vi "总磷总氮量程写入.vi"(7 "error in (no error)":errorcluster caption="错误输入（无错误）", 9 "量程参数写入":T1, 10 "测量参数":enum16{"总磷", "总氮"}(ring)) -> (0 "error out":errorcluster caption="错误输出")   [LabVIEW 2016, in "斯坦道总磷.lvlib"]
panel:
  out "输出数组":u16[](array[numeric]) format="%04x"
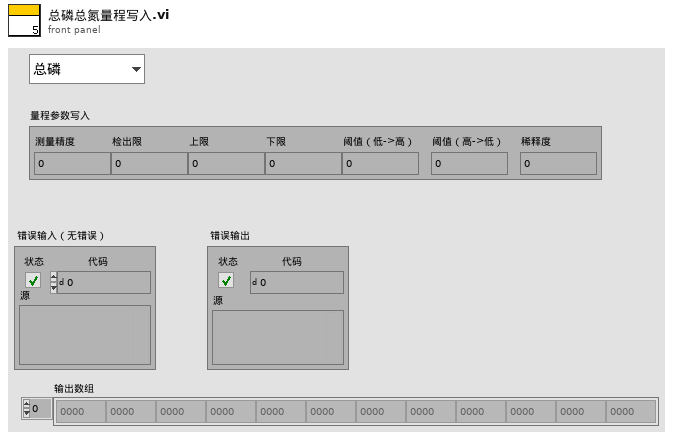
[diagram p1: front panel]
types:
  T1 = cluster{"测量精度":u16, "检出限":dbl, "上限":dbl, "下限":dbl, "阈值（低->高）":dbl, "阈值（高->低）":dbl, "稀释度":dbl}
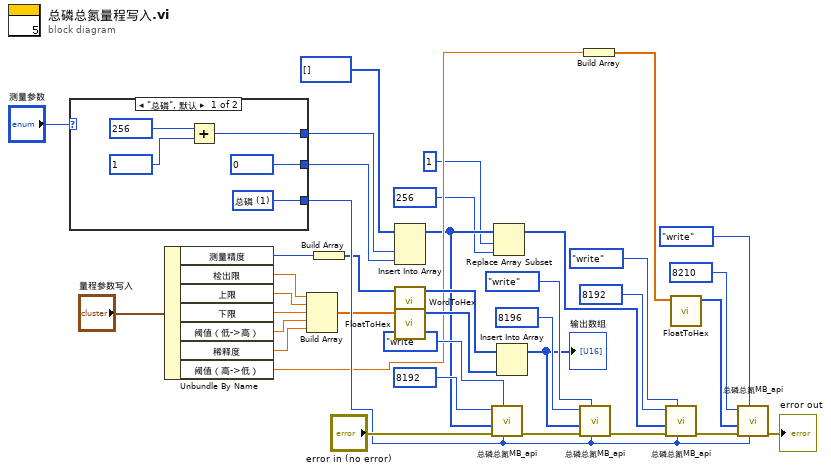
[diagram p0: block diagram]
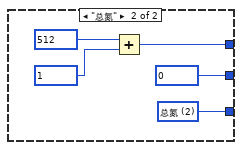
[diagram p2: hidden frame]
diagram:
  n1 = case shown="\"总磷\", 默认" "测量参数" {
    tunnel: [w38 w47] -> w21
    tunnel: [w39 w43] -> w5
    tunnel: [u16 0 ("starting address") u16 0 ("starting address")] -> w34
    frame "总磷", Default {
      w38 = u16 1 items=["总磷"=1, "总氮"=2, "氨氮"=3] ("站号")
      n2 = Add(x=u16 256 ("starting address"), y=u16 1 ("starting address")) -> (x+y=w39:u16)
    }
    frame "总氮" {
      w47 = u16 2 items=["总磷"=1, "总氮"=2, "氨氮"=3] ("站号")
      n3 = Add(x=u16 512 ("starting address"), y=u16 1 ("starting address")) -> (x+y=w43:u16)
    }
  }
  n4 = Unbundle By Name("量程参数写入") -> ("测量精度"=w18:u16, "检出限"=w17:dbl, "上限"=w16:dbl, "下限"=w15:dbl, "阈值（低->高）"=w14:dbl, "稀释度"=w13:dbl, "阈值（高->低）"=w8:dbl)
  n5 = Build Array(w17, w16, w15, w14, w13) -> (w12:dbl[])
  n6 = Build Array(w18) -> (w19:u16[])
  n7 = Insert Into Array(array=u16[] [] ("数组"), new element #1=w5, new element #2=w34) -> (w4:u16[])  [unwired: 1 in]
  n8 = call "WordToHex.vi"("WORD"=w19) -> ("数组"=w11:u16[])  [unwired: 10 in]
  n9 = call "FloatToHex.vi"("浮点数"=w12) -> ("DCBA整形输出"=w10:u16[])  [unwired: 10 in]
  n10 = call "总磷总氮MB_api.vi"("Slave ID"=w21, "STEP"=enum16{"open", "read", "write", "close"}."write", "Error in"="error in (no error)", "values"=w4, "starting address"=u16 8192) -> ("error out"=w31:errorcluster)  [unwired: 3 in, 3 out]
  n11 = Replace Array Subset(array=w4, new element=u16 256 ("starting address"), index=1 ("索引")) -> (w2:u16[])
  n12 = Insert Into Array(array=w11, new element=w10) -> (w9:u16[])  [unwired: 1 in]
  "输出数组" <- w9
  n13 = call "总磷总氮MB_api.vi"("Slave ID"=w21, "STEP"=enum16{"open", "read", "write", "close"}."write", "Error in"=w31, "values"=w9, "starting address"=u16 8196) -> ("error out"=w28:errorcluster)  [unwired: 3 in, 3 out]
  n14 = Build Array(w8) -> (w7:dbl[])
  n15 = call "总磷总氮MB_api.vi"("Slave ID"=w21, "STEP"=enum16{"open", "read", "write", "close"}."write", "Error in"=w28, "values"=w2, "starting address"=u16 8192) -> ("error out"=w27:errorcluster)  [unwired: 3 in, 3 out]
  n16 = call "FloatToHex.vi"("浮点数"=w7) -> ("DCBA整形输出"=w6:u16[])  [unwired: 10 in]
  n17 = call "总磷总氮MB_api.vi"("Slave ID"=w21, "STEP"=enum16{"open", "read", "write", "close"}."write", "Error in"=w27, "values"=w6, "starting address"=u16 8210) -> ("error out"=→"error out":errorcluster)  [unwired: 3 in, 3 out]
